vi "GDSAPI_CloneClass.vi"(8 "error in (no error)":errorcluster, 9 "NewClassPath(*.lvclass)":path, 10 "OriginalClassPath(*.lvclass)":path) -> (0 "error out":errorcluster)   [LabVIEW 2012]
doc: "Clone class\nThis VI clones the original class to a new class.\nMake sure the new class is located in a new folder."
uses:
  <resource>/Framework/Providers/Open_GDS/ClassProviders/Provider_LvNativeClass/ClassWriterNative_class/ClassWriterNative.lvclass
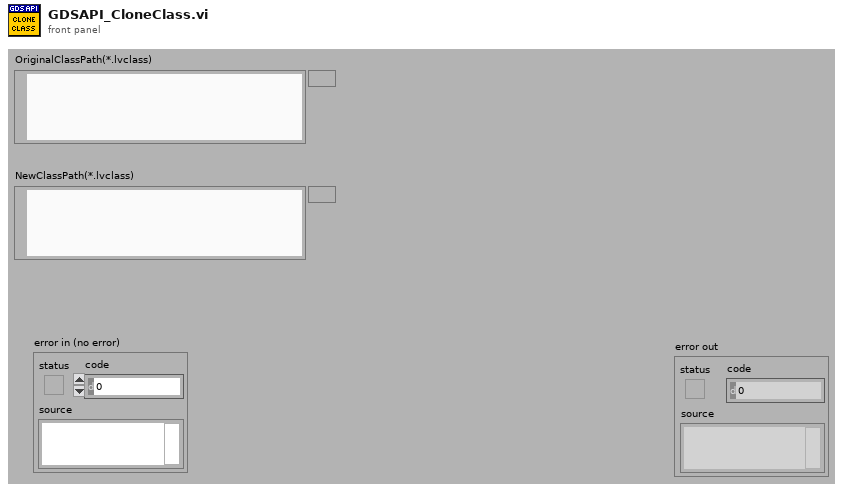
[diagram p1: front panel]
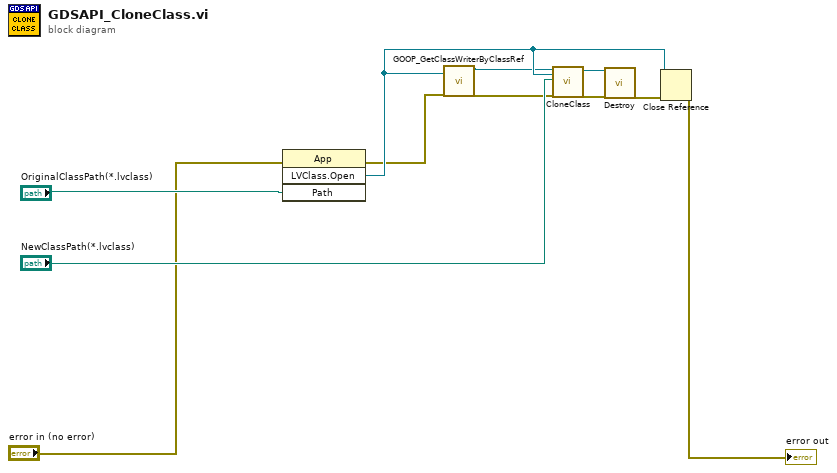
[diagram p0: block diagram]
diagram:
  n1 = invoke class="App" method="LVClass.Open"(error in="error in (no error)", "Path"="OriginalClassPath(*.lvclass)") -> (error out=w3:errorcluster, "LVClass.Open"=w4:refnum<vi>)  [unwired: 2 in, 2 out]
  n2 = call <resource>:"GOOP_GetClassWriterByClassRef.vi"("LVClassLibrary Refnum"=w4, "error in (no error)"=w3) -> ("ClassWriterNative.lvclass"=w2:refnum<class "ClassWriterNative.lvclass">, "error out"=w1:errorcluster)  [unwired: 16 in]
  n3 = call-dynamic "CloneClass.vi"("ClassWriterNative.lvclass"=w2, "ClassRef"=w4, "NewClassPath"="NewClassPath(*.lvclass)", "error in (no error)"=w1) -> ("ClassWriterNative.lvclass"=w7:refnum<class "ClassWriterNative.lvclass">, "error out"=w6:errorcluster)  [unwired: 13 in, 1 out]
  n4 = call-dynamic "Destroy.vi"("ClassWriterNative"=w7, "error in (no error)"=w6) -> ("error out"=w5:errorcluster)  [unwired: 17 in]
  n5 = Close Reference(reference=w4, error in (no error)=w5) -> (error out=→"error out":errorcluster)
